vi "Servo MSMT GSM Create Evaluations.vi"(8 "error in (no error)":errorcluster, 11 "Servo MSMT in":refnum<class "Servo MSMT.lvclass">) -> (0 "error out":errorcluster, 2 "GSM Evaluations":T1[](array[typedef]) {"Low Limit" format="%#_13g"; "SI Scaling" items=["femto"=-15, "pico"=-12, "nano"=-9, "micro"=-6, "milli"=-3, "percent"=-2, ""=0, "kilo"=3, "mega"=6, "giga"=9, "tera"=12]}, 3 "Servo MSMT out":refnum<class "Servo MSMT.lvclass">)   [LabVIEW 2018, in "Servo MSMT.lvlib" / "Servo MSMT.lvclass"]
uses:
  Servo MSMT.lvclass
  C:/Sequence Automation/Plugins/Measurement Interface.lvlibp/Measurement Interface.lvclass
  Plugins/TestStand API Tools (TSAT).lvlibp/Evaluation Actions/Includes/Controls/TSAT Evaluation.ctl
  Plugins/TestStand API Tools (TSAT).lvlibp/Evaluation Actions/Includes/Controls/TSAT Eval SI Unit Scaling.ctl
  Plugins/TestStand API Tools (TSAT).lvlibp/Evaluation Actions/Includes/Controls/TSAT Evaluation Type.ctl
  Servo MSMT.lvclass/Servo MSMT.ctl
  Plugins/SeqAuto IEvaluation.lvlibp/SeqAuto IEvaluation.lvclass
  Protected Methods/Read DC Pins.vi
  Protected Methods/Read Servo Measurements.vi
  Plugins/SeqAuto Evaluations.lvlibp/GSM Evaluations/Custom ORFS/GSM_ORFS_Custom.lvclass
  C:/Sequence Automation/Plugins/SeqAuto IEvaluation.lvlibp/SeqAuto IEvaluation.lvclass
  Plugins/SeqAuto Evaluations.lvlibp/GSM Evaluations/ModAcc/GSM_ModAcc.lvclass
  Plugins/SeqAuto Evaluations.lvlibp/GSM Evaluations/PFER/GSM_PFER.lvclass
  Plugins/SeqAuto Evaluations.lvlibp/GSM Evaluations/PVT/GSM_PVT.lvclass
  Plugins/SeqAuto Evaluations.lvlibp/Servo/Servo Gain/Servo Gain.lvclass
  Plugins/SeqAuto Evaluations.lvlibp/PA Evaluations/PAE/PAE.lvclass
  Plugins/SeqAuto Evaluations.lvlibp/DC Evaluations/DC_IDD.lvclass
  Plugins/Measurement Interface.lvlibp/Private Methods/Measurement Name/Read Measurement Name.vi
  Plugins/Measurement Interface.lvlibp/Private Methods/Measurement Parameters/Read Measurement Parameters.vi
  Plugins/String Database.lvlibp/String Database.lvclass
  Plugins/TestStand API Tools (TSAT).lvlibp/Evaluation Actions/TSAT Evaluation Actions.lvlib
  Plugins/Test Number and Bin Generator.lvlibp/Test Number and Bin Generator/Test Number and Bin Generator.lvclass
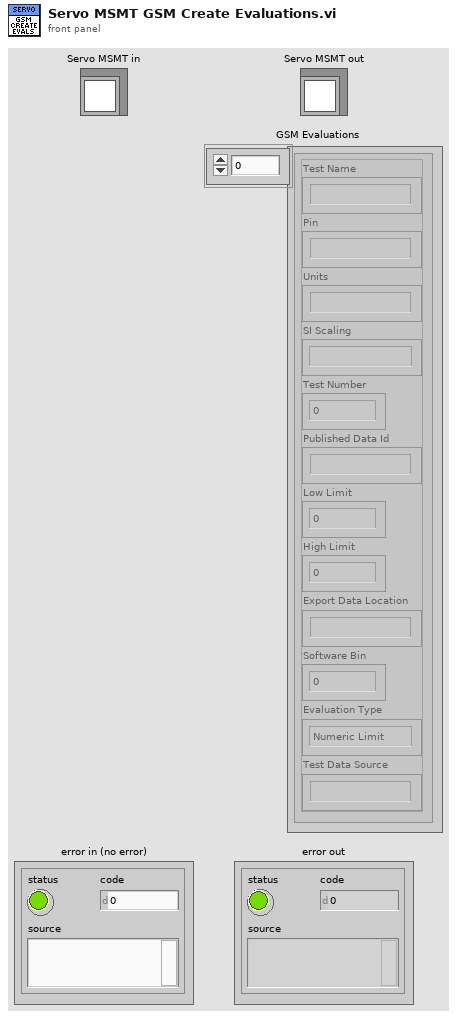
[diagram p1: front panel]
types:
  T1 = typedef "TestStand API Tools (TSAT).lvlibp/TSAT Evaluation Actions.lvlib/TSAT Evaluation.ctl" = cluster{"Test Name":string, "Pin":string, "Units":string, "SI Scaling":T2, "Test Number":i32, "Published Data Id":string, "Low Limit":dbl, "High Limit":dbl, "Export Data Location":string, "Software Bin":i64, "Evaluation Type":T3, "Test Data Source":string}
  T2 = typedef "TestStand API Tools (TSAT).lvlibp/TSAT Evaluation Actions.lvlib/TSAT Eval SI Unit Scaling.ctl" = i16
  T3 = typedef "TestStand API Tools (TSAT).lvlibp/TSAT Evaluation Actions.lvlib/TSAT Evaluation Type.ctl" = enum16{"Numeric Limit", "Pass/Fail", "None"}
  T4 = typedef "Test Number and Bin Generator.lvlibp/Test Number and Bin Generator.lvclass/Session Handle.ctl" = refnum<data-value>
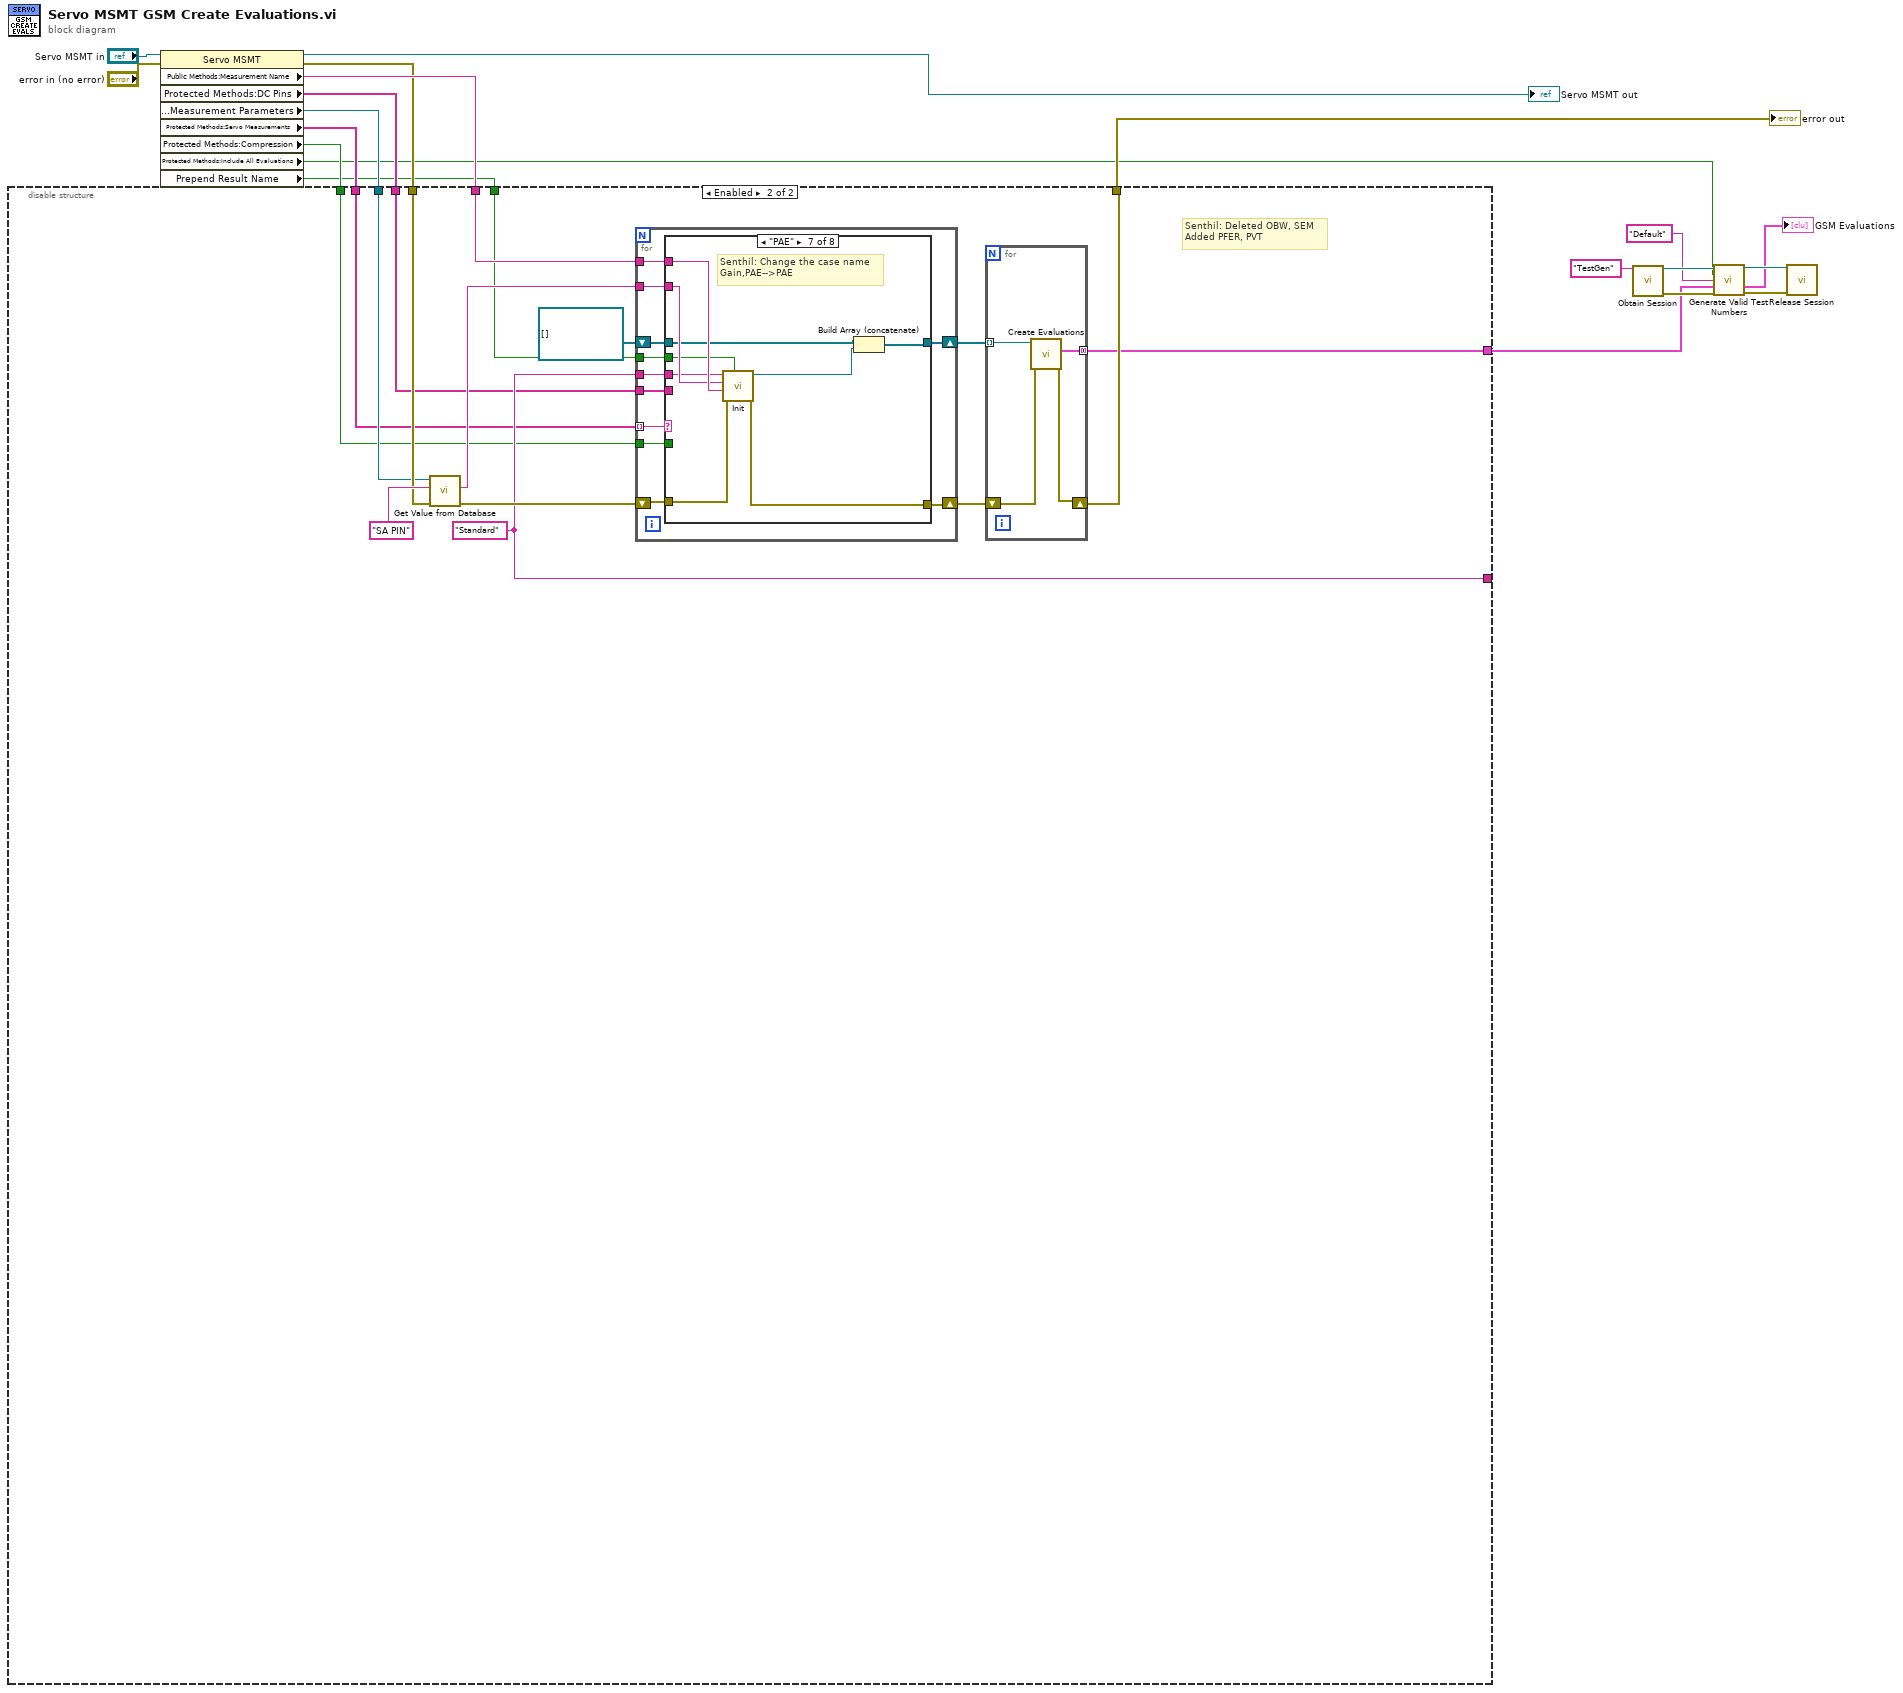
[diagram p0: block diagram]
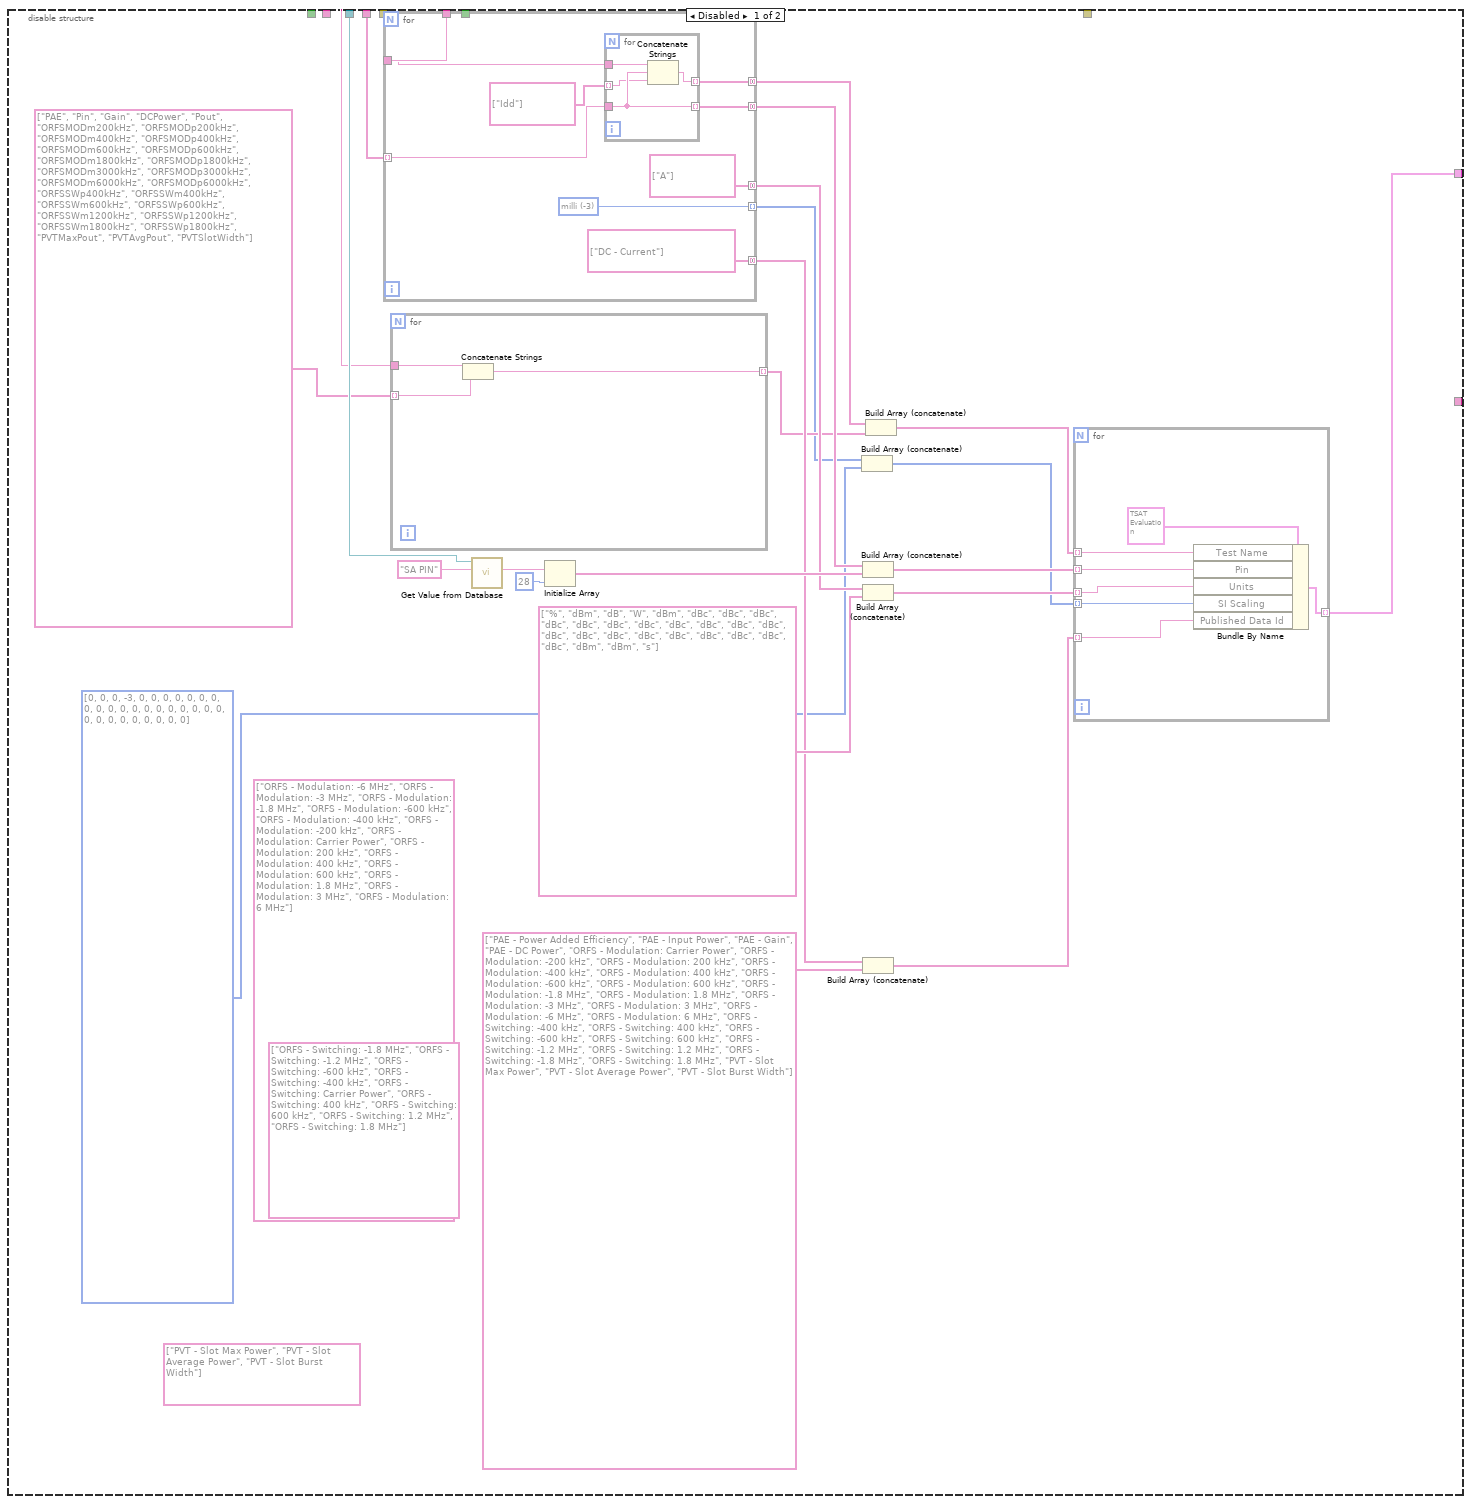
[diagram p2: hidden frame]
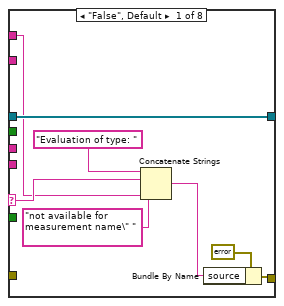
[diagram p3: hidden frame]
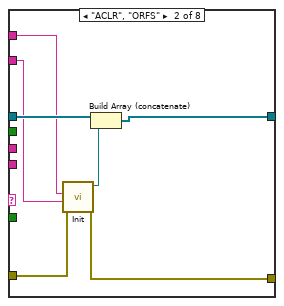
[diagram p4: hidden frame]
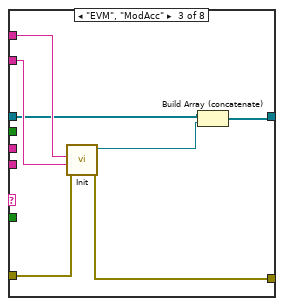
[diagram p5: hidden frame]
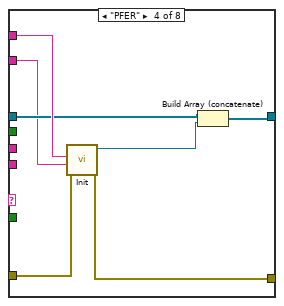
[diagram p6: hidden frame]
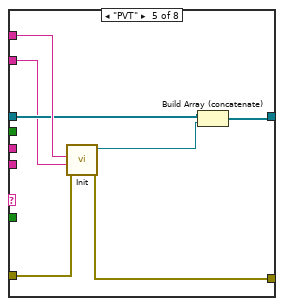
[diagram p7: hidden frame]
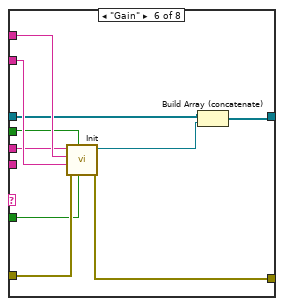
[diagram p8: hidden frame]
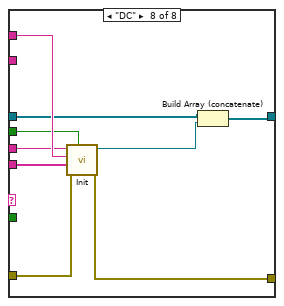
[diagram p9: hidden frame]
diagram:
  n1 = property class="Servo MSMT"(reference="Servo MSMT in", error in="error in (no error)") -> (reference out=→"Servo MSMT out":refnum<class "Servo MSMT.lvclass">, error out=w7:errorcluster, "Public Methods:Measurement Name"=w14:string, "Protected Methods:DC Pins"=w17:string[], "Protected Methods:Measurement Parameters"=w16:refnum<class "String Database.lvclass">, "Protected Methods:Servo Measurements"=w5:string[], "Protected Methods:Compression"=w4:bool, "Protected Methods:Include All Evaluations"=w2:bool, "Prepend Result Name"=w1:bool)
  n2 = disable-structure shown="Enabled" {
    disable-tunnel: w17 -> [w43 w70]
    disable-tunnel: w16 -> [w41 w69]
    disable-tunnel: w14 -> [w26 w75]
    disable-tunnel: [w21 w73] -> w8
    disable-tunnel: w7 -> [_ w71]
    disable-tunnel: [_ w74] -> w6
    disable-tunnel: [_ w72] -> _
    disable-tunnel: w5 -> [_ w68]
    disable-tunnel: w4 -> [_ w67]
    disable-tunnel: w1 -> [_ w66]
    frame Disabled {
      (unwired) string[] ["PVT - Slot Max Power", "PVT - Slot Average Power", "PVT - Slot Burst Width"]
      (unwired) string[] ["ORFS - Switching: -1.8 MHz", "ORFS - Switching: -1.2 MHz", "ORFS - Switching: -600 kHz", "ORFS - Switching: -400 kHz", "ORFS - Switching: Carrier Power", "ORFS - Switching: 400 kHz", "ORFS - Switching: 600 kHz", "ORFS - Switching: 1.2 MHz", "ORFS - Switching: 1.8 MHz"] ("Array")
      (unwired) string[] ["ORFS - Modulation: -6 MHz", "ORFS - Modulation: -3 MHz", "ORFS - Modulation: -1.8 MHz", "ORFS - Modulation: -600 kHz", "ORFS - Modulation: -400 kHz", "ORFS - Modulation: -200 kHz", "ORFS - Modulation: Carrier Power", "ORFS - Modulation: 200 kHz", "ORFS - Modulation: 400 kHz", "ORFS - Modulation: 600 kHz", "ORFS - Modulation: 1.8 MHz", "ORFS - Modulation: 3 MHz", "ORFS - Modulation: 6 MHz"] ("Array")
      w22 = T2[] [0, 0, 0, -3, 0, 0, 0, 0, 0, 0, 0, 0, 0, 0, 0, 0, 0, 0, 0, 0, 0, 0, 0, 0, 0, 0, 0, 0, 0, 0, 0, 0] items=["femto"=-15, "pico"=-12, "nano"=-9, "micro"=-6, "milli"=-3, "percent"=-2, ""=0, "kilo"=3, "mega"=6, "giga"=9, "tera"=12]
      n3 = for {
        tunnel: w43 -> [w51] mode=indexing
        tunnel: w26 -> [w48]
        tunnel: [w53] -> w42 mode=concatenating
        tunnel: [string[] ["A"]] -> w33 mode=concatenating
        tunnel: [w50] -> w37 mode=concatenating
        tunnel: [string[] ["DC - Current"]] -> w31 mode=concatenating
        tunnel: [w47] -> w24 mode=indexing
        w47 = T2 -3 items=["femto"=-15, "pico"=-12, "nano"=-9, "micro"=-6, "milli"=-3, "percent"=-2, ""=0, "kilo"=3, "mega"=6, "giga"=9, "tera"=12] ("SI Scaling")
        n4 = for {
          tunnel: w48 -> [w58]
          tunnel: string[] ["Idd"] -> [w55] mode=indexing
          tunnel: [w57] -> w53 mode=indexing
          tunnel: w51 -> [w56]
          tunnel: [w56] -> w50 mode=indexing
          n5 = Concatenate Strings(w58, w56, w55) -> (w57:string)
        }
      }
      n6 = for {
        tunnel: string[] ["PAE", "Pin", "Gain", "DCPower", "Pout", "ORFSMODm200kHz", "ORFSMODp200kHz", "ORFSMODm400kHz", "ORFSMODp400kHz", "ORFSMODm600kHz", "ORFSMODp600kHz", "ORFSMODm1800kHz", "ORFSMODp1800kHz", "ORFSMODm3000kHz", "ORFSMODp3000kHz", "ORFSMODm6000kHz", "ORFSMODp6000kHz", "ORFSSWp400kHz", "ORFSSWm400kHz", "ORFSSWm600kHz", "ORFSSWp600kHz", "ORFSSWm1200kHz", "ORFSSWp1200kHz", "ORFSSWm1800kHz", "ORFSSWp1800kHz", "PVTMaxPout", "PVTAvgPout", "PVTSlotWidth"] -> [w45] mode=indexing
        tunnel: w26 -> [w46]
        tunnel: [w44] -> w25 mode=indexing
        n7 = Concatenate Strings(w46, w45) -> (w44:string)
      }
      n8 = call "Get Value from Database.vi"("Entry Name"="SA PIN", "Message in"=w41) -> ("Entry Value"=w38:string)  [unwired: 6 in, 3 out]
      n9 = Initialize Array(w38, 28) -> (w36:string[])
      n10 = Build Array (concatenate)(w24, w22) -> (w23:T2[])
      n11 = Build Array (concatenate)(w37, w36) -> (w35:string[])
      n12 = Build Array (concatenate)(w33, string[] ["%", "dBm", "dB", "W", "dBm", "dBc", "dBc", "dBc", "dBc", "dBc", "dBc", "dBc", "dBc", "dBc", "dBc", "dBc", "dBc", "dBc", "dBc", "dBc", "dBc", "dBc", "dBc", "dBc", "dBc", "dBm", "dBm", "s"]) -> (w32:string[])
      n13 = Build Array (concatenate)(w31, string[] ["PAE - Power Added Efficiency", "PAE - Input Power", "PAE - Gain", "PAE - DC Power", "ORFS - Modulation: Carrier Power", "ORFS - Modulation: -200 kHz", "ORFS - Modulation: 200 kHz", "ORFS - Modulation: -400 kHz", "ORFS - Modulation: 400 kHz", "ORFS - Modulation: -600 kHz", "ORFS - Modulation: 600 kHz", "ORFS - Modulation: -1.8 MHz", "ORFS - Modulation: 1.8 MHz", "ORFS - Modulation: -3 MHz", "ORFS - Modulation: 3 MHz", "ORFS - Modulation: -6 MHz", "ORFS - Modulation: 6 MHz", "ORFS - Switching: -400 kHz", "ORFS - Switching: 400 kHz", "ORFS - Switching: -600 kHz", "ORFS - Switching: 600 kHz", "ORFS - Switching: -1.2 MHz", "ORFS - Switching: 1.2 MHz", "ORFS - Switching: -1.8 MHz", "ORFS - Switching: 1.8 MHz", "PVT - Slot Max Power", "PVT - Slot Average Power", "PVT - Slot Burst Width"]) -> (w29:string[])
      n14 = Build Array (concatenate)(w42, w25) -> (w28:string[])
      n15 = for {
        tunnel: w28 -> [w64] mode=indexing
        tunnel: [w63] -> w21 mode=indexing
        tunnel: w35 -> [w62] mode=indexing
        tunnel: w32 -> [w61] mode=indexing
        tunnel: w29 -> [w60] mode=indexing
        tunnel: w23 -> [w59] mode=indexing
        n16 = Bundle By Name(cluster=T1 {"Test Name"="test", "Pin"="test", "Units"="dB", "SI Scaling"=-9, "Test Number"=0, "Published Data Id"="test", "Low Limit"=-999999.0, "High Limit"=999999.0, "Export Data Location"="", "Software Bin"=-1, "Evaluation Type"=enum."Numeric Limit", "Test Data Source"=""} ("Evaluation"), "Test Name"=w64, "Pin"=w62, "Units"=w61, "SI Scaling"=w59, "Published Data Id"=w60) -> (w63:T1)
      }
    }
    frame Enabled {
      w72 = "Standard" ("Entry Name")
      # "Senthil: Deleted OBW, SEM\nAdded PFER, PVT"
      n17 = call "Get Value from Database.vi"("error in (no error)"=w71, "Entry Name"="SA PIN", "Message in"=w69) -> ("error out"=w80:errorcluster, "Entry Value"=w76:string)  [unwired: 5 in, 2 out]
      n18 = for {
        tunnel: w76 -> [w96]
        tunnel: w75 -> [w95]
        shift-right: [w93] -> w79
        shift-left: refnum<class "SeqAuto IEvaluation.lvclass">[] [] -> [w94]
        tunnel: w68 -> [w92] mode=indexing
        shift-right: [w90] -> w77
        shift-left: w80 -> [w91]
        tunnel: w70 -> [w89]
        tunnel: w72 -> [w88]
        tunnel: w67 -> [w87]
        tunnel: w66 -> [w86]
        n19 = case shown="\"PAE\"" w92 {
          selector: w92 -> [w100 _ _ _ _ _ _ _]
          tunnel: w96 -> [_ w105 w117 w119 w126 w141 w150 _]
          tunnel: w95 -> [w98 w106 w118 w125 w132 w142 w151 w160]
          tunnel: [w104 w111 w112 w120 w127 w136 w145 w155] -> w93
          tunnel: w94 -> [w104 w110 w114 w122 w129 w138 w147 w157]
          tunnel: w91 -> [_ w108 w116 w124 w131 w140 w149 w159]
          tunnel: [w102 w107 w115 w123 w130 w139 w148 w158] -> w90
          tunnel: w89 -> [_ _ _ _ _ _ _ w154]
          tunnel: w88 -> [_ _ _ _ _ w135 w144 w153]
          tunnel: w87 -> [_ _ _ _ _ w134 _ _]
          tunnel: w86 -> [_ _ _ _ _ w133 w143 w152]
          frame "False", Default {
            n20 = Concatenate Strings("Evaluation of type: " ("source"), w100, "not available for measurement name\" " ("source"), w98) -> (w97:string)
            n21 = Bundle By Name(cluster=errorcluster {"status"=TRUE, "code"=7777, "source"=""} ("error out"), "source"=w97) -> (w102:errorcluster)
          }
          frame "ACLR", "ORFS" {
            n22 = call "Init.vi"("error in (no error)"=w108, "SA Pin"=w105, "Measurement Name"=w106) -> ("error out"=w107:errorcluster, "GSM_ORFS_Custom out"=w109:refnum<class "GSM_ORFS_Custom.lvclass">)  [unwired: 7 in]
            n23 = Build Array (concatenate)(w110, w109) -> (w111:refnum<class "SeqAuto IEvaluation.lvclass">[])
          }
          frame "EVM", "ModAcc" {
            n24 = call "Init.vi"("error in (no error)"=w116, "SA Pin"=w117, "Measurement Name"=w118) -> ("error out"=w115:errorcluster, "GSM_ModAcc_out"=w113:refnum<class "GSM_ModAcc.lvclass">)  [unwired: 7 in]
            n25 = Build Array (concatenate)(w114, w113) -> (w112:refnum<class "SeqAuto IEvaluation.lvclass">[])
          }
          frame "PFER" {
            n26 = call "Init.vi"("error in (no error)"=w124, "SA Pin"=w119, "Measurement Name"=w125) -> ("error out"=w123:errorcluster, "GSM_PFER_out"=w121:refnum<class "GSM_PFER.lvclass">)  [unwired: 7 in]
            n27 = Build Array (concatenate)(w122, w121) -> (w120:refnum<class "SeqAuto IEvaluation.lvclass">[])
          }
          frame "PVT" {
            n28 = call "Init.vi"("error in (no error)"=w131, "SA Pin"=w126, "Measurement Name"=w132) -> ("error out"=w130:errorcluster, "GSM_PVT_out"=w128:refnum<class "GSM_PVT.lvclass">)  [unwired: 7 in]
            n29 = Build Array (concatenate)(w129, w128) -> (w127:refnum<class "SeqAuto IEvaluation.lvclass">[])
          }
          frame "Gain" {
            n30 = call "Init.vi"("Compression?"=w134, "Prepend Result Name"=w133, "error in (no error)"=w140, "SA Pin"=w141, "Measurement Name"=w142, "Standard"=w135) -> ("error out"=w139:errorcluster, "Servo Gain out"=w137:refnum<class "Servo Gain.lvclass">)  [unwired: 4 in]
            n31 = Build Array (concatenate)(w138, w137) -> (w136:refnum<class "SeqAuto IEvaluation.lvclass">[])
          }
          frame "PAE" {
            # "Senthil: Change the case name\nGain,PAE-->PAE"
            n32 = call "Init.vi"("Prepend Result Name"=w143, "error in (no error)"=w149, "Measurement Name"=w151, "SA Pin"=w150, "Standard"=w144) -> ("error out"=w148:errorcluster, "PAE out"=w146:refnum<class "PAE.lvclass">)  [unwired: 5 in]
            n33 = Build Array (concatenate)(w147, w146) -> (w145:refnum<class "SeqAuto IEvaluation.lvclass">[])
          }
          frame "DC" {
            n34 = call "Init.vi"("Prepend Result Name"=w152, "error in (no error)"=w159, "DC Pins"=w154, "Measurement Name"=w160, "Standard"=w153) -> ("error out"=w158:errorcluster, "DC_IDD out"=w156:refnum<class "DC_IDD.lvclass">)  [unwired: 5 in]
            n35 = Build Array (concatenate)(w157, w156) -> (w155:refnum<class "SeqAuto IEvaluation.lvclass">[])
          }
        }
      }
      n36 = for {
        tunnel: w79 -> [w85] mode=indexing
        tunnel: [w84] -> w73 mode=concatenating
        shift-right: [w82] -> w74
        shift-left: w77 -> [w83]
        n37 = call-dynamic "Create Evaluations.vi"("error in (no error)"=w83, "IEvaluation in"=w85) -> ("error out"=w82:errorcluster, "Evaluations Out"=w84:T1[])  [unwired: 7 in, 1 out]
      }
    }
  }
  "error out" <- w6
  n38 = call "Obtain Session.vi"("Session  Name ()"="TestGen") -> ("Session Handle"=w13:T4, "error out"=w11:errorcluster)  [unwired: 13 in]
  n39 = call "Generate Valid Test Numbers.vi"("Session Handle in"=w13, "Include All Evaluations?"=w2, "Test Group"="Default", "Evaluations In"=w8, "error in (no error)"=w11) -> ("Session Handle out"=w12:T4, "Evaluations Out"=→"GSM Evaluations":T1[], "error out"=w10:errorcluster)  [unwired: 8 in]
  n40 = call "Release Session.vi"("Session Handle"=w12, "error in (no error)"=w10) -> ()  [unwired: 13 in, 1 out]
